vi "MGI SZL New Zip File.vi"(8 "Error In":errorcluster, 9 "Confirm Overwrite? (F)":bool, 11 "Target Path":path) -> (0 "Error Out":errorcluster, 1 "Cancelled?":bool, 3 "New Zip File":refnum<k24>)   [LabVIEW 2020]
doc: "Creates a new empty zip file in the path specified by target path. The new file overwrties an existing file or produces an overwrite confirmation dialog based on the value of confirm overwrite?.\n\nThis VI relies on the Sharp Zip Library which is a .NET assembly written in C# by Mike Krueger. It is licenced under the GPL with a special exception permitting independent modules to link to the library regardless of the license terms of the independent module. \n\nMore information about the library and its license is available from:\nhttp://www.icsharpcode.net/opensource/sharpziplib/\n\nAuthored by Matthew G. Harrison\nsupport@mooregoodideas.com\nwww.mooregoodideas.com\n\nCopyright (c) 2010, Moore Good Ideas, Inc.\n\nAll rights reserved.\n\nRedistribution and use in source and binary forms, with or without modification, are permitted provided that the following conditions are met:\n\n * Redistributions of source code must retain the above copyright notice, this list of conditions and the following disclaimer.\n * Redistributions in binary form must reproduce the above copyright notice, this list of conditions and the following disclaimer in the documentation and/or other materials provided with the distribution.\n * Neither the name of Moore Good Ideas, Inc. nor the names of its contributors may be used to endorse or promote products derived from this software without specific prior written permission.\n\nTHIS SOFTWARE IS PROVIDED BY THE COPYRIGHT HOLDERS AND CONTRIBUTORS \"AS IS\" AND ANY EXPRESS OR IMPLIED WARRANTIES, INCLUDING, BUT NOT LIMITED TO, THE IMPLIED WARRANTIES OF MERCHANTABILITY AND FITNESS FOR A PARTICULAR PURPOSE ARE DISCLAIMED. IN NO EVENT SHALL THE COPYRIGHT OWNER OR CONTRIBUTORS BE LIABLE FOR ANY DIRECT, INDIRECT, INCIDENTAL, SPECIAL, EXEMPLARY, OR CONSEQUENTIAL DAMAGES (INCLUDING, BUT NOT LIMITED TO, PROCUREMENT OF SUBSTITUTE GOODS OR SERVICES; LOSS OF USE, DATA, OR PROFITS; OR BUSINESS INTERRUPTION) HOWEVER CAUSED AND ON ANY THEORY OF LIABILITY, WHETHER IN CONTRACT, STRICT LIABILITY, OR TORT (INCLUDING NEGLIGENCE OR OTHERWISE) ARISING IN ANY WAY OUT OF THE USE OF THIS SOFTWARE, EVEN IF ADVISED OF THE POSSIBILITY OF SUCH DAMAGE."
uses:
  C:/Program Files/National Instruments/LabVIEW 2020/user.lib/_MGI/File/Zip/Support Files/ICSharpCode.SharpZipLib.dll
  Support Files/ICSharpCode.SharpZipLib.dll
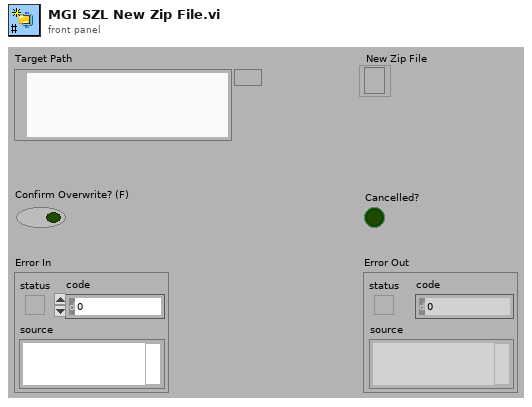
[diagram p1: front panel]
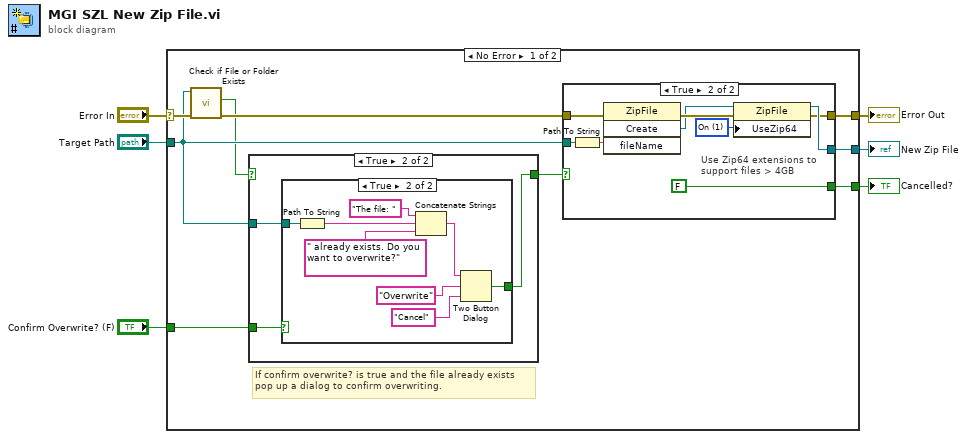
[diagram p0: block diagram]
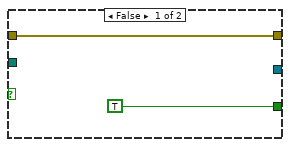
[diagram p2: hidden frame]
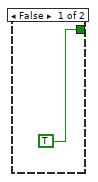
[diagram p3: hidden frame]
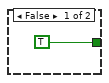
[diagram p4: hidden frame]
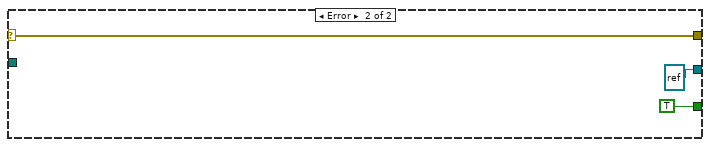
[diagram p5: hidden frame]
diagram:
  n1 = case shown="No Error" "Error In" {
    selector: "Error In" -> [w10 w42]
    tunnel: "Confirm Overwrite? (F)" -> [w15 _]
    tunnel: [w13 TRUE ("cancelled")] -> w5
    tunnel: [w12 refnum<k24> refnum ("Create")] -> w4
    tunnel: [w11 w42] -> w3
    tunnel: "Target Path" -> [w8 _]
    frame No Error {
      # "If confirm overwrite? is true and the file already exists\npop up a dialog to confirm overwriting."
      n2 = call <vilib>:"Check if File or Folder Exists.vi"("error in (no error)"=w10, "path"=w8) -> ("error out"=w9:errorcluster, "file or folder exists?"=w7:bool)  [unwired: 7 in, 1 out]
      n3 = case shown="True" w7 {
        tunnel: w8 -> [_ w29]
        tunnel: w15 -> [_ w30]
        tunnel: [TRUE ("T button?") w28] -> w14
        frame False {
        }
        frame True {
          n4 = case shown="True" w30 {
            tunnel: w29 -> [_ w35]
            tunnel: [TRUE ("T button?") w32] -> w28
            frame False {
            }
            frame True {
              n5 = Path To String(path=w35) -> (string=w34:string)
              n6 = Concatenate Strings("The file: " ("string"), w34, " already exists. Do you want to overwrite?" ("message")) -> (w33:string)
              n7 = Two Button Dialog(message=w33, 1:"Cancel" ("F button name (\"Cancel\")"), 2:"Overwrite" ("T button name (\"OK\")")) -> (T button?=w32:bool)
            }
          }
        }
      }
      n8 = case shown="True" w14 {
        tunnel: w8 -> [_ w25]
        tunnel: [TRUE ("cancelled") FALSE ("cancelled")] -> w13
        tunnel: w9 -> [w16 w23]
        tunnel: [_ w19] -> w12
        tunnel: [w16 w18] -> w11
        frame False {
        }
        frame True {
          w22 = 1 items=["Off", "On", "Dynamic"] ("UseZip64")
          # "Use Zip64 extensions to\nsupport files > 4GB"
          n9 = Path To String(path=w25) -> (string=w26:string)
          n10 = invoke class="ZipFile" method="Create"(error in=w23, "fileName"=w26) -> (error out=w21:errorcluster, "Create"=w20:refnum<k24>)  [unwired: 2 in, 2 out]
          n11 = property class="ZipFile"(reference=w20, error in=w21, "UseZip64"=w22) -> (reference out=w19:refnum<k24>, error out=w18:errorcluster)
        }
      }
    }
    frame Error {
    }
  }
  "Error Out" <- w3
  "Cancelled?" <- w5
  "New Zip File" <- w4
